vi "Clear Disabled Overlays.vi"(8 "error in":errorcluster, 10 "Disabled Overlays":string[](array[string]), 11 "BigMAQ in":refnum<class "BigMAQ.lvclass">) -> (0 "error out":errorcluster, 3 "BigMAQ out":refnum<class "BigMAQ.lvclass">)   [LabVIEW 2019, in "BigMAQ.lvclass"]
uses:
  BigMAQ.lvclass
  BigMAQ.lvclass/BigMAQ.ctl
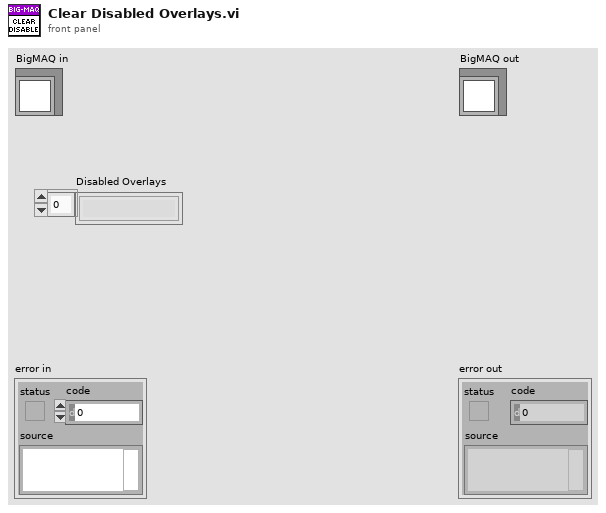
[diagram p1: front panel]
types:
  T1 = typedef "IMAQ Image.ctl" = refnum<image>
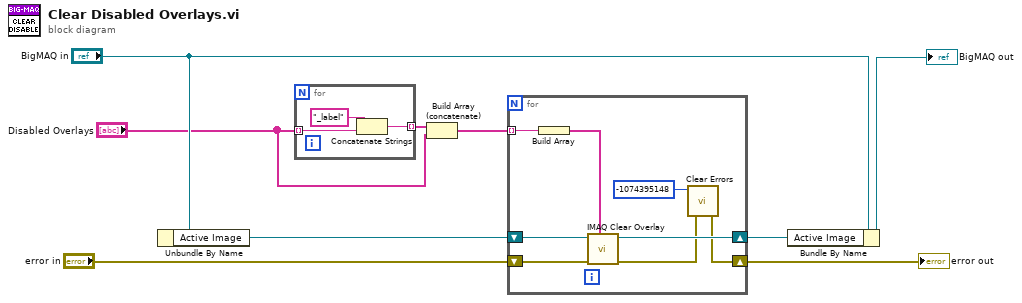
[diagram p0: block diagram]
diagram:
  n1 = Unbundle By Name("BigMAQ in") -> ("Active Image"=w9:T1)
  n2 = for {
    tunnel: "Disabled Overlays" -> [w12] mode=indexing
    tunnel: [w10] -> w5 mode=indexing
    n3 = Concatenate Strings("_label" ("string"), w12) -> (w10:string)
  }
  n4 = Build Array (concatenate)(w5, "Disabled Overlays") -> (w3:string[])
  n5 = for {
    tunnel: w3 -> [w16] mode=indexing
    shift-right: [w18] -> w2
    shift-left: w9 -> [w20]
    shift-right: [w14] -> w1
    shift-left: "error in" -> [w19]
    n6 = Build Array(w16) -> (w17:string[])
    n7 = call "IMAQ Clear Overlay"("Groups"=w17, "error in (no error)"=w19, "Image"=w20) -> ("error out"=w13:errorcluster, "Image Out"=w18:T1)  [unwired: 7 in]
    n8 = call <vilib>:"Clear Errors.vi"("error in (no error)"=w13, "specific error code to clear (0: all)"=-1074395148) -> ("error out"=w14:errorcluster)  [unwired: 4 in, 1 out]
  }
  "error out" <- w1
  n9 = Bundle By Name(cluster="BigMAQ in", "Active Image"=w2) -> (→"BigMAQ out":refnum<class "BigMAQ.lvclass">)
